vi "Encode DAQ Params.vi"(8 "error in (no error)":errorcluster, 11 "Data in":variant) -> (0 "error out":errorcluster, 3 "Data out":variant)   [LabVIEW 2026, in "TALOS.lvlib" / "Guardian.lvlib" / "Guardian.lvclass"]
uses:
  Guardian.lvclass
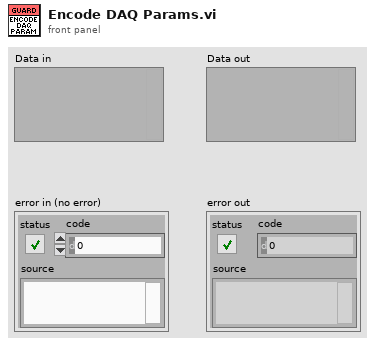
[diagram p1: front panel]
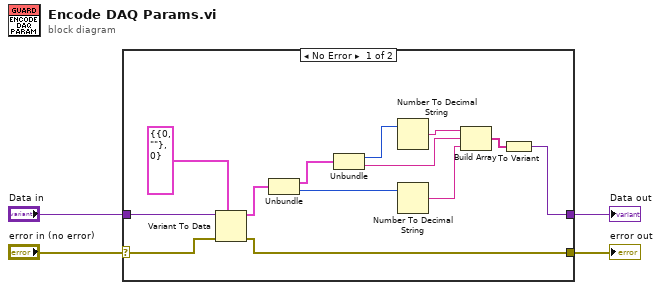
[diagram p0: block diagram]
diagram:
  n1 = case shown="No Error" "error in (no error)" {
    selector: "error in (no error)" -> [w17 w19]
    tunnel: "Data in" -> [w16 w18]
    tunnel: [w6 w18] -> w2
    tunnel: [w5 w19] -> w1
    frame No Error {
      n2 = Variant To Data(error in=w17, type=cluster{cluster{u16, string}, i32} {{0, ""}, 0}, Variant=w16) -> (data=w14:cluster{cluster{u16, string}, i32}, error out=w5:errorcluster)
      n3 = Unbundle(w14) -> (w13:cluster{u16, string}, w11:i32)
      n4 = Unbundle(w13) -> (w12:u16, w9:string)
      n5 = Number To Decimal String(number=w12) -> (decimal integer string=w10:string)  [unwired: 1 in]
      n6 = Number To Decimal String(number=w11) -> (decimal integer string=w8:string)  [unwired: 1 in]
      n7 = Build Array(w10, w9, w8) -> (w7:string[])
      n8 = To Variant(anything=w7) -> (Variant=w6:variant)
    }
    frame Error {
    }
  }
  "Data out" <- w2
  "error out" <- w1
